vi "CC Read Air Mass Data.vi"(8 "error in (no error)":errorcluster, 11 "file path (dialog if empty)":path) -> (0 "error out":errorcluster, 2 "Air Mass":T1[](array[typedef]), 3 "BlockIDs":string[](array[string]))   [LabVIEW 2021]
uses:
  CC cluster Air Mass Data.ctl
  <vilib>/Utility/file.llb/Read Delimited Spreadsheet (string).vi
panel:
  out "all rows":string[][](array[string])
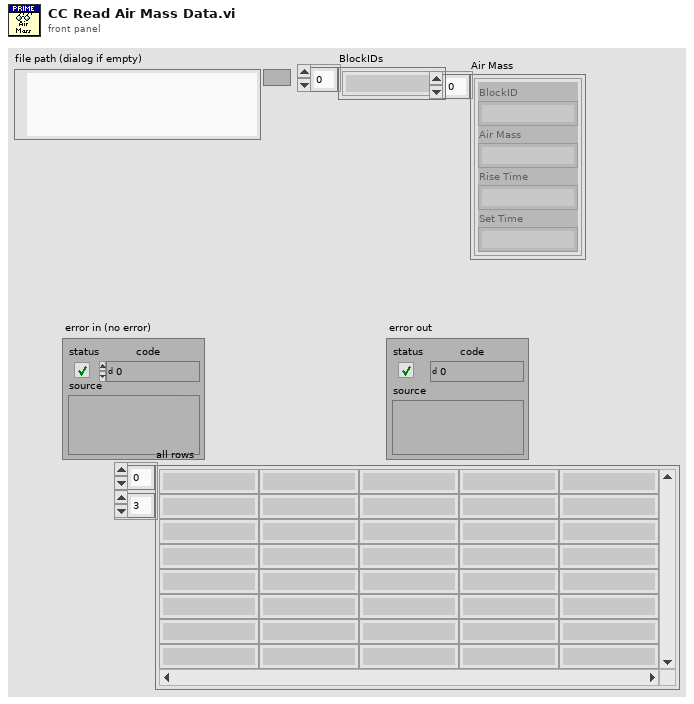
[diagram p1: front panel]
types:
  T1 = typedef "CC cluster Air Mass Data.ctl" = cluster{"BlockID":string, "Air Mass":string, "Rise Time":string, "Set Time":string}
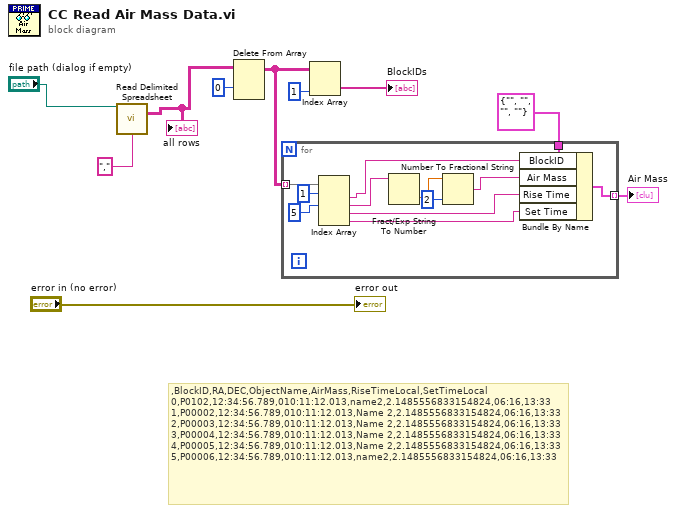
[diagram p0: block diagram]
diagram:
  # ",BlockID,RA,DEC,ObjectName,AirMass,RiseTimeLocal,SetTimeLocal\n0,P0102,12:34:56.789,010:11:12.013,name2,2.1485556833154824,06:16,13:33\n1,P00002,12:34:56.789,010:11:12.013,Name 2,2.1485556833154824,06:16,13:33\n2,P00003,12:34:56.789,010:11:12.013,Name 2,2.1485556833154824,06:16,13:33\n3,P00004,12:34:56.789,010:11:12.013,Name 2,2.1485556833154824,06:16,13:33\n4,P00005,12:34:56.789,010:11:12.013,Name 2,2.1485556833154824,06:16,13:33\n5,P00006,12:34:56.789,010:11:12.013,name2,2.1485556833154824,06:16,13:33"
  n1 = call-poly <vilib>:"Read Delimited Spreadsheet.vi"("file path (dialog if empty)"="file path (dialog if empty)", "delimiter (\\t)"="," ("delimiter (\\t)")) -> ("all rows"=w5:string[][])  [unwired: 8 in, 5 out]
  "all rows" <- w5
  n2 = Delete From Array(array=w5, index (row)=0) -> (array with subset deleted=w3:string[][])  [unwired: 2 in, 1 out]
  n3 = for {
    tunnel: w3 -> [w22] mode=indexing
    tunnel: T1 {"BlockID"="", "Air Mass"="", "Rise Time"="", "Set Time"=""} -> [w21]
    tunnel: [w20] -> w2 mode=indexing
    n4 = Index Array(array=w22, index #1=1 ("index"), index #2=5 ("index")) -> (element #1=w18:string, element #2=w14:string, element #3=w17:string, element #4=w16:string)  [unwired: 2 in]
    n5 = Fract/Exp String To Number(string=w14) -> (number=w13:dbl)  [unwired: 3 in, 1 out]
    n6 = Number To Fractional String(number=w13, precision (6)=i16 2) -> (F-format string=w11:string)  [unwired: 2 in]
    n7 = Bundle By Name(cluster=w21, "BlockID"=w18, "Air Mass"=w11, "Rise Time"=w17, "Set Time"=w16) -> (w20:T1)
  }
  "Air Mass" <- w2
  n8 = Index Array(array=w3, index (col)=1 ("disabled index (col)")) -> (element=→"BlockIDs":string[])  [unwired: 1 in]
  "error out" <- "error in (no error)"
